vi "Sequencer Main.vi"() -> ()   [LabVIEW 2018] (continued)
                                n2343 = To Lower Case(string=w4629) -> (all lower case string=w4628:string)
                              }
                              n2344 = Multiply(x=w4617, y=-0.2) -> (x*y=w4620:dbl)
                              n2345 = Bundle("Lower Limit"=w4617, "Upper Limit"=w4618, "Numeric Value"=w4625) -> (w4626:T36)  [unwired: 1 in]
                              n2346 = Multiply(x=w4618, y=0.2) -> (x*y=w4622:dbl)
                              n2347 = Add(x=w4620, y=w4617) -> (x+y=w4619:dbl)
                              n2348 = Add(x=w4622, y=w4618) -> (x+y=w4621:dbl)
                              n2349 = property on="Limits" class="Slide (strict)"("Value"=w4626) -> ()  [unwired: 2 in, 2 out]
                              n2350 = property on="Limits" class="Slide (strict)"("Scale.Maximum"=w4621, "Scale.Minimum"=w4619) -> ()  [unwired: 2 in, 2 out]
                              n2351 = Index Array(array=w4615, index #1=0 ("index"), index #2=1 ("index"), index #3=2 ("index"), index #4=3 ("index"), index #5=4 ("index")) -> (element #1=w4614:string, element #2=w4608:string, element #3=w4607:string, element #4=w4606:string, element #5=w4605:string)
                            }
                            frame #1 {
                              n2352 = Not Equal?(x=w4648, y=4) -> (x != y?=w4640:bool)
                              n2353 = case shown="\"on\"" w4653 {
                                tunnel: w4652 -> [_ w4673]
                                tunnel: w4651 -> [_ w4672]
                                tunnel: w4650 -> [_ w4671]
                                tunnel: w4649 -> [_ w4670]
                                tunnel: [10000.0 w4661] -> w4642
                                tunnel: [w4655 w4660] -> w4646
                                tunnel: [w4654 w4659] -> w4645
                                tunnel: [w4654 w4658] -> w4644
                                tunnel: w4640 -> [_ w4657]
                                frame "off", Default {
                                w4654 = 0
                                w4655 = i16 0 items=["Sine"=0, "Square"=1, "Triangle"=2, "Ramp Up"=3, "Ramp Down"=4, "DC"=8, "Arbitrary"=6] ("Wave Type")
                                }
                                frame "on" {
                                w4664 = 1000000
                                n2354 = case shown="True" w4657 {
                                frame False {
                                }
                                frame True {
                                n2355 = One Button Dialog(message="PICo Scoê parameters\nErr!") -> ()  [unwired: 1 in, 1 out]
                                }
                                }
                                n2356 = Scan From String(input string=w4672) -> (output 1=w4667:dbl)  [unwired: 4 in, 3 out]
                                n2357 = Scan From String(input string=w4671) -> (output 1=w4666:dbl)  [unwired: 4 in, 3 out]
                                n2358 = Scan From String(input string=w4670) -> (output 1=w4665:dbl)  [unwired: 4 in, 3 out]
                                n2359 = Multiply(x=w4666, y=w4664) -> (x*y=w4663:dbl)
                                n2360 = Multiply(x=w4665, y=w4664) -> (x*y=w4662:dbl)
                                n2361 = To Long Integer(number=w4663) -> (32bit integer=w4659:i32)
                                n2362 = To Long Integer(number=w4662) -> (32bit integer=w4658:i32)
                                n2363 = case shown="\"triangle\"" w4673 {
                                tunnel: [w4677 w4678 w4679 w4680] -> w4660
                                frame "sine", Default {
                                w4677 = i16 0 items=["Sine"=0, "Square"=1, "Triangle"=2, "Ramp Up"=3, "Ramp Down"=4, "DC"=8, "Arbitrary"=6] ("Wave Type")
                                }
                                frame "square" {
                                w4678 = i16 1 items=["Sine"=0, "Square"=1, "Triangle"=2, "Ramp Up"=3, "Ramp Down"=4, "DC"=8, "Arbitrary"=6] ("Wave Type")
                                }
                                frame "triangle" {
                                w4679 = i16 2 items=["Sine"=0, "Square"=1, "Triangle"=2, "Ramp Up"=3, "Ramp Down"=4, "DC"=8, "Arbitrary"=6] ("Wave Type")
                                }
                                frame "dc" {
                                w4680 = i16 8 items=["Sine"=0, "Square"=1, "Triangle"=2, "Ramp Up"=3, "Ramp Down"=4, "DC"=8, "Arbitrary"=6] ("Wave Type")
                                }
                                }
                                n2364 = Greater Or Equal?(x=w4667, y=50000.0) -> (x >= y?=w4668:bool)
                                n2365 = case shown="True" w4668 {
                                tunnel: [w4675 50000.0] -> w4661
                                tunnel: w4667 -> [w4675 _]
                                frame False {
                                }
                                frame True {
                                }
                                }
                                }
                              }
                              n2366 = Bundle By Name(cluster=T29 {"Peak-to-Peak Voltage (microvolts)"=1000000, "Offset Voltage (microvolts)"=0, "Wave Type"=0, "Sweep Type"=0, "Shots"=0, "Sweeps"=0, "Trigger Type"=0, "Trigger Source"=0, "Ext. Threshold (ADC count)"=0, "White Noise"=FALSE} ("General AWG Settings"), "Wave Type"=w4646, "Peak-to-Peak Voltage (microvolts)"=w4645, "Offset Voltage (microvolts)"=w4644) -> (w4637:T29)
                              n2367 = global read "Global Variable.vi" "PicoScope Handle"() -> (w4638:u32)
                              n2368 = Bundle By Name(cluster=T30 {"Start Frequency"=1000.0, "Stop Frequency"=1000.0, "Increment"=0.0, "Dwell Time (seconds)"=0.0} ("Standard Waveform Settings"), "Start Frequency"=w4642, "Stop Frequency"=w4642) -> (w4639:T30)
                              n2369 = call "PicoScope3000aAWG.vi"("Standard Waveform Settings"=w4639, "General AWG Settings"=w4637, "Handle In"=w4638) -> ("error out"=w4636:errorcluster)  [unwired: 5 in, 3 out]
                              n2370 = call "PicoErrorHandler.vi"("error in"=w4636) -> ("error out"=w4635:errorcluster)
                              n2371 = call <userlib>:"Clear All Errors__ogtk.vi"("Error In"=w4635) -> ()  [unwired: 3 in, 1 out]
                            }
                          }
                          n2372 = Unbundle By Name(w4586) -> ("status"=w4584:bool)
                          n2373 = Not(x=w4584) -> (.not. x?=w4585:bool)
                          n2374 = case shown="True" w4585 {
                            tunnel: [enum16{"Idle", "PASS", "FALSE"}."FALSE" ("Step Test Result") enum16{"Idle", "PASS", "FALSE"}."PASS" ("Step Test Result")] -> w4592
                            frame False {
                            }
                            frame True {
                            }
                          }
                        }
                        frame 60 {
                          w4697 = "------------------------" ("string")
                          w4696 = "\r\n"
                          # "Step TEST Result"
                          # "Step Result Msg"
                          # "Str with \"false\" goto parameters"
                          # "Str \"false\" Preset"
                          # "Cmd Case"
                          # "Cmd Case"
                          n2375 = Unbundle By Name(w4710) -> ("Parameters"=w4692:string, "Step Description"=w4681:string, "Test Values.Numeric Value"=w4686:dbl, "Test Values.Upper Limit"=w4685:dbl, "Test Values.Lower Limit"=w4684:dbl)
                          n2376 = in-place {
                            in-place-border: w4692 -> [w4742]
                            in-place-border: [w4741] -> w4691
                            in-place-border: [w4740] -> w4689
                            # "STr \"fase\" exist"
                            n2377 = To Lower Case(string=w4742) -> (all lower case string=w4743:string)
                            n2378 = Match Pattern(string=w4743, regular expression="false") -> (after substring=w4745:string, offset past match=w4746:i32)  [unwired: 1 in, 2 out]
                            n2379 = Greater Or Equal To 0?(x=w4746) -> (x >= 0?=w4740:bool)
                            n2380 = case shown="True" w4740 {
                              tunnel: w4745 -> [_ w4749]
                              tunnel: [string[] [] w4748] -> w4741
                              frame False {
                                (unwired) ""
                              }
                              frame True {
                                n2381 = while {
                                shift-right: [w4753] -> _
                                shift-left: w4749 -> [w4754]
                                tunnel: [w4750] -> w4748 mode=indexing
                                stop <- w4752 stop-if-true
                                # "Get Array of Sub Parametrs"
                                n2382 = Match Pattern(string=w4754, regular expression=":") -> (before substring=w4750:string, after substring=w4753:string, offset past match=w4751:i32)  [unwired: 1 in, 1 out]
                                n2383 = Less Than 0?(x=w4751) -> (x < 0?=w4752:bool)
                                }
                              }
                            }
                          }
                          n2384 = while {
                            shift-right: [w4759] -> _
                            shift-left: w4692 -> [w4760]
                            tunnel: [w4756] -> w4694 mode=indexing
                            stop <- w4758 stop-if-true
                            # "Get Array of Parametrs"
                            n2385 = Match Pattern(string=w4760, regular expression=">") -> (before substring=w4756:string, after substring=w4759:string, offset past match=w4757:i32)  [unwired: 1 in, 1 out]
                            n2386 = Less Than 0?(x=w4757) -> (x < 0?=w4758:bool)
                          }
                          n2387 = Concatenate Strings(w4681, w4696, w4697, w4697, w4697, w4696) -> (w4698:string)
                          n2388 = property on="Tab Control Msg" class="TabCtl (strict)"("Value"=T21."Serial" ("Tab Control Msg")) -> (error out=w4708:errorcluster)  [unwired: 2 in, 1 out]
                          n2389 = property on="Serial CMD Mon" class="Str"("Value"=w4698) -> ()  [unwired: 2 in, 2 out]
                          n2390 = Index Array(array=w4694, index=0) -> (element=w4706:string)
                          n2391 = Index Array(array=w4694, index=1) -> (element=w4704:string)
                          n2392 = Index Array(array=w4694, index=2) -> (element=w4701:string)
                          n2393 = Index Array(array=w4694, index=3) -> (element=w4699:string)
                          n2394 = Index Array(array=w4694, index=4) -> (element=w4693:string)
                          n2395 = case shown="\"enable_ble\"" w4706 {
                            tunnel: w4708 -> [_ _ _ _ _ _ _ _ _ _ _ _ _ _ _ _ _ _ _ _]
                            tunnel: [enum16{"Idle", "PASS", "FALSE"}."FALSE" ("Step Test Result") w4770 w4814 w4842 w4885 w4935 w5079 w5119 w5165 w5343 w5414 w5573 w5623 w5672 w5708 w5745 w5782 w5814 w5846 w5878] -> w4707
                            tunnel: w4704 -> [_ w4768 _ _ _ w4947 w5083 w5117 _ w5341 w5440 _ _ w5673 _ w5746 _ _ w5844 _]
                            tunnel: w4701 -> [_ _ _ _ _ w4946 w5082 _ _ w5329 w5439 _ _ _ _ _ _ _ _ _]
                            tunnel: w4699 -> [_ _ _ _ _ w4945 w5081 _ _ _ _ _ _ _ _ _ _ _ _ _]
                            tunnel: w4693 -> [_ _ _ _ _ w4944 w5080 _ _ _ _ _ _ _ _ _ _ _ _ _]
                            tunnel: ["" w4767 w4811 w4840 w4876 w4934 w5078 w5115 w5163 w5328 w5434 "Set capmem '1' then '0' " w5622 w5671 _ _ w5780 w5812 _ _] -> w4683
                            tunnel: w4686 -> [_ _ _ _ _ _ _ _ _ _ _ _ _ _ _ _ _ _ _ _]
                            tunnel: w4685 -> [_ _ _ _ _ _ _ _ _ _ _ _ w5629 _ _ _ _ _ _ _]
                            tunnel: w4684 -> [_ _ _ _ _ _ _ _ _ _ _ _ w5628 _ _ _ _ _ _ _]
                            tunnel: ["" w4766 w4813 w4839 w4875 w4933 w5077 w5114 w5162 w5320 w5413 w5571 w5620 w5670 w5707 w5744 w5779 w5811 w5843 w5877] -> w4682
                            frame "False", Default {
                              n2396 = One Button Dialog(message="!Sequencer File Err") -> ()  [unwired: 1 in, 1 out]
                            }
                            frame "open" {
                              # "Param"
                              # "Cmd"
                              n2397 = flat-sequence {
                                tunnel: [w4782] -> w4772
                                tunnel: [w4781] -> w4771
                                tunnel: [w4780] -> w4769
                                tunnel: w4772 -> [w4788]
                                tunnel: w4771 -> [w4793]
                                tunnel: [w4794] -> w4770
                                tunnel: w4769 -> [w4791]
                                tunnel: w4768 -> [w4790]
                                tunnel: [w4792] -> w4767
                                tunnel: [w4791] -> w4766
                                frame #0 {
                                w4773 = u16 2 items=["None", "XON/XOFF", "RTS/CTS", "XON/XOFF & RTS/CTS", "DTR/DSR", "XON/XOFF & DTR/DSR"] ("flow control (0:none)")
                                n2398 = global read "Global Variable.vi" "COM Port FTDI RS232"() -> (w4779:refnum<visa-resource-name>)
                                n2399 = call "ADB-Serial_WrRd.vi"("flow control (0:none)"=w4773, "Tx Deay"=u16 5, "Timeout(Sec)"=2.0, "PassString"="Chuck(1)", "Command"="open", "ComPort"=w4779) -> ("error out"=w4781:errorcluster, "PASS"=w4782:bool, "received"=w4780:string)  [unwired: 3 in]
                                n2400 = invoke on="Serial CMD Mon" class="Str" method="Append String"("string"=w4780) -> ()  [unwired: 3 in, 4 out]
                                n2401 = Wait (ms)(milliseconds to wait=u32 500) -> ()  [unwired: 1 out]
                                }
                                frame #1 {
                                n2402 = String Length(string=w4790) -> (length=w4789:i32)
                                n2403 = Equal To 0?(x=w4789) -> (x = 0?=w4784:bool)
                                n2404 = Not(x=w4784) -> (.not. x?=w4783:bool)
                                n2405 = case shown="True" w4788 {
                                tunnel: w4791 -> [_ w4803]
                                tunnel: w4790 -> [_ w4807]
                                tunnel: [FALSE w4804] -> w4786
                                tunnel: ["!Firmware vertion not Right" ("line") w4802] -> w4792
                                frame False {
                                }
                                frame True {
                                n2406 = To Lower Case(string=w4807) -> (all lower case string=w4806:string)
                                n2407 = To Lower Case(string=w4803) -> (all lower case string=w4808:string)
                                n2408 = Match Pattern(string=w4808, regular expression=w4806) -> (match substring=w4800:string, offset past match=w4805:i32)  [unwired: 1 in, 2 out]
                                n2409 = Greater Than 0?(x=w4805) -> (x > 0?=w4804:bool)
                                n2410 = Concatenate Strings("version: ", w4800) -> (w4802:string)
                                }
                                }
                                n2411 = And(x=w4788, y=w4784) -> (x .and. y?=w4785:bool)
                                n2412 = global read "Global Variable.vi" "Array Errors"() -> (w4797:errorcluster[])
                                n2413 = Replace Array Subset(array=w4797, new element=w4793, index=3) -> (w4796:errorcluster[])
                                n2414 = global write "Global Variable.vi" "Array Errors"(w4796) -> ()
                                n2415 = Select(t=w4786, s=w4783, f=w4785) -> (s? t:f=w4787:bool)
                                n2416 = case shown="True" w4787 {
                                tunnel: [enum16{"Idle", "PASS", "FALSE"}."FALSE" ("Step Test Result") enum16{"Idle", "PASS", "FALSE"}."PASS" ("Step Test Result")] -> w4794
                                frame False {
                                # "Step TEST Result"
                                }
                                frame True {
                                # "Step TEST Result"
                                }
                                }
                                }
                              }
                            }
                            frame "passwd" {
                              n2417 = flat-sequence {
                                tunnel: [w4826] -> w4816
                                tunnel: [w4825] -> w4815
                                tunnel: [w4824] -> w4812
                                tunnel: w4816 -> [w4829]
                                tunnel: w4815 -> [w4830]
                                tunnel: [w4831] -> w4814
                                tunnel: [w4828] -> w4813
                                tunnel: w4812 -> [w4828]
                                tunnel: [w4827] -> w4811
                                frame #0 {
                                w4817 = u16 2 items=["None", "XON/XOFF", "RTS/CTS", "XON/XOFF & RTS/CTS", "DTR/DSR", "XON/XOFF & DTR/DSR"] ("flow control (0:none)")
                                n2418 = global read "Global Variable.vi" "COM Port FTDI RS232"() -> (w4823:refnum<visa-resource-name>)
                                n2419 = call "ADB-Serial_WrRd.vi"("flow control (0:none)"=w4817, "Tx Deay"=u16 5, "Timeout(Sec)"=2.0, "PassString"="Chuck(3)", "Command"="passwd admin", "ComPort"=w4823) -> ("error out"=w4825:errorcluster, "PASS"=w4826:bool, "received"=w4824:string)  [unwired: 3 in]
                                n2420 = invoke on="Serial CMD Mon" class="Str" method="Append String"("string"=w4824) -> ()  [unwired: 3 in, 4 out]
                                n2421 = Wait (ms)(milliseconds to wait=u32 250) -> ()  [unwired: 1 out]
                                }
                                frame #1 {
                                n2422 = global read "Global Variable.vi" "Array Errors"() -> (w4834:errorcluster[])
                                n2423 = case shown="False" w4829 {
                                tunnel: [enum16{"Idle", "PASS", "FALSE"}."FALSE" ("Step Test Result") enum16{"Idle", "PASS", "FALSE"}."PASS" ("Step Test Result")] -> w4831
                                tunnel: ["Err" "Admin"] -> w4827
                                frame False {
                                # "Step TEST Result"
                                }
                                frame True {
                                # "Step TEST Result"
                                }
                                }
                                n2424 = Replace Array Subset(array=w4834, new element=w4830, index=3) -> (w4833:errorcluster[])
                                n2425 = global write "Global Variable.vi" "Array Errors"(w4833) -> ()
                                }
                              }
                            }
                            frame "getpid" {
                              # "Param"
                              # "Cmd"
                              n2426 = flat-sequence {
                                tunnel: [w4854] -> w4844
                                tunnel: [w4853] -> w4843
                                tunnel: [w4852] -> w4841
                                tunnel: [w4852] -> _
                                tunnel: [w4852] -> w4839
                                tunnel: w4844 -> [w4858]
                                tunnel: w4843 -> [w4861]
                                tunnel: [w4862] -> w4842
                                tunnel: [w4855] -> w4840
                                tunnel: w4841 -> [w4859]
                                frame #0 {
                                w4845 = u16 2 items=["None", "XON/XOFF", "RTS/CTS", "XON/XOFF & RTS/CTS", "DTR/DSR", "XON/XOFF & DTR/DSR"] ("flow control (0:none)")
                                n2427 = global read "Global Variable.vi" "COM Port FTDI RS232"() -> (w4851:refnum<visa-resource-name>)
                                n2428 = global read "Global Variable.vi" "Wr PID"() -> (w4848:string)
                                n2429 = call "ADB-Serial_WrRd.vi"("flow control (0:none)"=w4845, "Tx Deay"=u16 5, "Timeout(Sec)"=2.0, "PassString"=w4848, "Command"="getPID", "ComPort"=w4851) -> ("error out"=w4853:errorcluster, "PASS"=w4854:bool, "received"=w4852:string)  [unwired: 3 in]
                                n2430 = invoke on="Serial CMD Mon" class="Str" method="Append String"("string"=w4852) -> ()  [unwired: 3 in, 4 out]
                                n2431 = Wait (ms)(milliseconds to wait=u32 250) -> ()  [unwired: 1 out]
                                }
                                frame #1 {
                                n2432 = in-place {
                                in-place-border: w4861 -> [w4869]
                                in-place-border: [w4869] -> w4860
                                in-place-border: [w4870] -> w4856
                                in-place-border: w4859 -> [w4867]
                                n2433 = Match Pattern(string=w4867, regular expression="PID:" ("search string/char (-)")) -> (after substring=w4866:string)  [unwired: 1 in, 3 out]
                                n2434 = String Subset(string=w4866, offset (0)=1, length (rest)=13 ("length (rest)")) -> (substring=w4870:string)
                                n2435 = global write "Global Variable.vi" "Rd PID"(w4870) -> ()
                                }
                                n2436 = global read "Global Variable.vi" "Array Errors"() -> (w4865:errorcluster[])
                                n2437 = case shown="False" w4858 {
                                tunnel: [enum16{"Idle", "PASS", "FALSE"}."FALSE" ("Step Test Result") enum16{"Idle", "PASS", "FALSE"}."PASS" ("Step Test Result")] -> w4862
                                frame False {
                                # "Step TEST Result"
                                }
                                frame True {
                                # "Step TEST Result"
                                }
                                }
                                n2438 = Replace Array Subset(array=w4865, new element=w4860, index=3) -> (w4864:errorcluster[])
                                n2439 = global write "Global Variable.vi" "Array Errors"(w4864) -> ()
                                n2440 = Concatenate Strings("Read PID: " ("string"), w4856) -> (w4855:string)
                                }
                              }
                            }
                            frame "setpid" {
                              n2441 = flat-sequence {
                                tunnel: [w4888] -> w4879
                                tunnel: [w4930] -> w4881
                                tunnel: [w4929] -> w4880
                                tunnel: w4879 -> [w4924]
                                tunnel: [w4926] -> w4877
                                tunnel: [w4925] -> w4875
                                frame #0 {
                                w4899 = 5
                                # "Replace Space to 0"
                                # "YY: Year 00-99\nWW: Week 01-53\nSS: Supplier ID (SVI: 04)\nxx: Spare\nNNNNN: Ser Number"
                                # "default"
                                n2442 = local read "Barcode"() -> (w4887:string)
                                n2443 = global write "Global Variable.vi" "Wr PID"("") -> ()
                                n2444 = String Length(string=w4887) -> (length=w4898:i32)
                                n2445 = Greater?(x=w4898, y=w4899) -> (0:w4900:bool)
                                n2446 = case shown="True" w4900 {
                                tunnel: w4887 -> [_ w4923]
                                tunnel: w4899 -> [_ w4921]
                                tunnel: w4898 -> [_ w4922]
                                tunnel: "1111040011111" ("ADB_PID") -> [w4903 w4919]
                                tunnel: [w4903 w4909] -> w4893
                                frame False {
                                }
                                frame True {
                                w4905 = "%2d" ("format string")
                                n2447 = Subtract(x=w4922, y=w4921) -> (x-y=w4920:i32)
                                n2448 = call "Calc_ISO_WeekNumber.vi"() -> ("ISO week number"=w4904:i32, "SBZ year 2 digits"=w4908:i32)  [unwired: 5 in, 5 out]
                                n2449 = String Subset(string=w4923, offset (0)=w4920, length (rest)=w4921) -> (substring=w4918:string)
                                n2450 = Format Into String(format string=w4905, w4908) -> (resulting string=w4907:string)  [unwired: 2 in, 1 out]
                                n2451 = Replace Substring(2:5 ("length (len. of substring)"), 3:8 ("offset (0)"), 4:w4918, 5:w4919) -> (1:w4915:string)  [unwired: 1 out]
                                n2452 = Format Into String(format string=w4905, w4904) -> (resulting string=w4906:string)  [unwired: 2 in, 1 out]
                                n2453 = Replace Substring(2:2 ("offset (0)"), 3:0 ("offset (0)"), 4:w4907, 5:w4915) -> (1:w4910:string)  [unwired: 1 out]
                                n2454 = Replace Substring(2:2 ("offset (0)"), 3:2 ("offset (0)"), 4:w4906, 5:w4910) -> (1:w4909:string)  [unwired: 1 out]
                                }
                                }
                                n2455 = local read "Barcode\nDefault"() -> (w4886:bool)
                                n2456 = call <vilib>:"Space Constant.vi"() -> ("String"=w4891:string)
                                n2457 = call <vilib>:"Search and Replace Pattern.vi"("string"=w4893, "regular expression (\"\")"=w4891, "replace string (\"\")"="0" ("replace string (\"\")")) -> ("result string"=w4889:string)  [unwired: 2 in, 1 out]
                                n2458 = case shown="False" w4886 {
                                tunnel: w4889 -> [_ w4902]
                                tunnel: [w4901 w4902] -> w4888
                                tunnel: w4887 -> [w4901 _]
                                frame False {
                                }
                                frame True {
                                }
                                }
                                n2459 = Concatenate Strings("Calculated PID: ", w4888, "\r\n") -> (w4890:string)
                                n2460 = invoke on="Serial CMD Mon" class="Str" method="Append String"("string"=w4890) -> ()  [unwired: 3 in, 4 out]
                                }
                                frame #1 {
                                n2461 = global read "Global Variable.vi" "COM Port FTDI RS232"() -> (w4928:refnum<visa-resource-name>)
                                n2462 = call "ADB-SetPID.vi"("ADB_PID"=w4924, "ComPort"=w4928) -> ("error out"=w4929:errorcluster, "Wr PID"=w4926:string, "PASS"=w4930:bool, "received"=w4925:string)  [unwired: 6 in]
                                n2463 = invoke on="Serial CMD Mon" class="Str" method="Append String"("string"=w4925) -> ()  [unwired: 3 in, 4 out]
                                n2464 = global write "Global Variable.vi" "Wr PID"(w4926) -> ()
                                n2465 = Wait (ms)(milliseconds to wait=u32 5000) -> ()  [unwired: 1 out]
                                }
                              }
                              n2466 = global read "Global Variable.vi" "Array Errors"() -> (w4884:errorcluster[])
                              n2467 = case shown="False" w4881 {
                                tunnel: [enum16{"Idle", "PASS", "FALSE"}."FALSE" ("Step Test Result") enum16{"Idle", "PASS", "FALSE"}."PASS" ("Step Test Result")] -> w4885
                                frame False {
                                # "Step TEST Result"
                                }
                                frame True {
                                # "Step TEST Result"
                                }
                              }
                              n2468 = Replace Array Subset(array=w4884, new element=w4880, index=5) -> (w4883:errorcluster[])
                              n2469 = Concatenate Strings("Write PID: " ("string"), w4877) -> (w4876:string)
                              n2470 = global write "Global Variable.vi" "Array Errors"(w4883) -> ()
                            }
                            frame "recvtest" {
                              # "Param 1-4"
                              # "Cmd"
                              n2471 = flat-sequence {
                                tunnel: [w4966] -> w4950
                                tunnel: [w4965] -> w4949
                                tunnel: [w4964] -> w4948
                                tunnel: w4947 -> [w4963]
                                tunnel: w4946 -> [w4962]
                                tunnel: w4945 -> [w4961]
                                tunnel: w4944 -> [w4960]
                                tunnel: [w4959] -> w4943
                                tunnel: [w4958] -> w4942
                                tunnel: [w4957] -> w4941
                                tunnel: [w4956] -> w4940
                                tunnel: [w4955] -> w4939
                                tunnel: [w4954] -> w4938
                                tunnel: [w4953] -> w4937
                                tunnel: [w4952] -> w4936
                                tunnel: w4950 -> [w5005]
                                tunnel: w4949 -> [w5024]
                                tunnel: [w5025] -> w4935
                                tunnel: w4948 -> [w5003]
                                tunnel: w4943 -> [w5015]
                                tunnel: w4942 -> [w5014]
                                tunnel: w4941 -> [w5013]
                                tunnel: w4940 -> [w5012]
                                tunnel: w4939 -> [w5011]
                                tunnel: w4938 -> [w5010]
                                tunnel: w4937 -> [w5009]
                                tunnel: w4936 -> [w5008]
                                tunnel: [w5004] -> w4934
                                tunnel: [w5003] -> w4933
                                frame #0 {
                                w4951 = "%f" ("format string")
                                n2472 = for {
                                N: 1 -> [_]
                                tunnel: [w4999] -> w4966
                                tunnel: [w4998] -> w4965
                                tunnel: [w4997] -> w4964
                                stop <- w4999 stop-if-true
                                n2473 = global read "Global Variable.vi" "COM Port FTDI RS232"() -> (w5002:refnum<visa-resource-name>)
                                n2474 = call "ADB-Serial_WrRd.vi"("Timeout(Sec)"=5.0, "PassString"="Chuck(3):", "Command"="recvtest", "ComPort"=w5002) -> ("error out"=w4998:errorcluster, "PASS"=w4999:bool, "received"=w4997:string)  [unwired: 5 in]
                                n2475 = invoke on="Serial CMD Mon" class="Str" method="Append String"("string"=w4997) -> ()  [unwired: 3 in, 4 out]
                                }
                                n2476 = in-place {
                                in-place-border: w4963 -> [w4995]
                                in-place-border: [w4991] -> w4959
                                in-place-border: [w4990] -> w4958
                                in-place-border: w4951 -> [w4989]
                                # "max"
                                # "min"
                                # "LMS RX -> k_est"
                                n2477 = Match Pattern(string=w4995, regular expression=":") -> (before substring=w4993:string, after substring=w4992:string)  [unwired: 1 in, 2 out]
                                n2478 = Scan From String(format string=w4989, input string=w4993) -> (output 1=w4991:dbl)  [unwired: 3 in, 3 out]
                                n2479 = Scan From String(format string=w4989, input string=w4992) -> (output 1=w4990:dbl)  [unwired: 3 in, 3 out]
                                }
                                n2480 = in-place {
                                in-place-border: w4962 -> [w4988]
                                in-place-border: [w4984] -> w4957
                                in-place-border: [w4983] -> w4956
                                in-place-border: w4951 -> [w4982]
                                # "max"
                                # "min"
                                # "LMS RX -> I_est"
                                n2481 = Match Pattern(string=w4988, regular expression=":") -> (before substring=w4986:string, after substring=w4985:string)  [unwired: 1 in, 2 out]
                                n2482 = Scan From String(format string=w4982, input string=w4986) -> (output 1=w4984:dbl)  [unwired: 3 in, 3 out]
                                n2483 = Scan From String(format string=w4982, input string=w4985) -> (output 1=w4983:dbl)  [unwired: 3 in, 3 out]
                                }
                                n2484 = in-place {
                                in-place-border: w4961 -> [w4981]
                                in-place-border: [w4977] -> w4955
                                in-place-border: [w4976] -> w4954
                                in-place-border: w4951 -> [w4975]
                                # "max"
                                # "min"
                                # "CURRENT -> k_est"
                                n2485 = Match Pattern(string=w4981, regular expression=":") -> (before substring=w4979:string, after substring=w4978:string)  [unwired: 1 in, 2 out]
                                n2486 = Scan From String(format string=w4975, input string=w4979) -> (output 1=w4977:dbl)  [unwired: 3 in, 3 out]
                                n2487 = Scan From String(format string=w4975, input string=w4978) -> (output 1=w4976:dbl)  [unwired: 3 in, 3 out]
                                }
                                n2488 = in-place {
                                in-place-border: w4960 -> [w4974]
                                in-place-border: [w4971] -> w4953
                                in-place-border: [w4970] -> w4952
                                in-place-border: w4951 -> [w4969]
                                # "max"
                                # "min"
                                # "CURRENT -> I_est"
                                n2489 = Match Pattern(string=w4974, regular expression=":") -> (before substring=w4973:string, after substring=w4972:string)  [unwired: 1 in, 2 out]
                                n2490 = Scan From String(format string=w4969, input string=w4973) -> (output 1=w4971:dbl)  [unwired: 3 in, 3 out]
                                n2491 = Scan From String(format string=w4969, input string=w4972) -> (output 1=w4970:dbl)  [unwired: 3 in, 3 out]
                                }
                                }
                                frame #1 {
                                n2492 = Match Pattern(string=w5003, regular expression="CURRENT:") -> (after substring=w5006:string, offset past match=w5020:i32)  [unwired: 1 in, 2 out]
                                n2493 = Match Pattern(string=w5003, regular expression="LMS_RX:") -> (after substring=w5007:string, offset past match=w5021:i32)  [unwired: 1 in, 2 out]
                                n2494 = Greater Than 0?(x=w5021) -> (x > 0?=w5018:bool)
                                n2495 = Greater Than 0?(x=w5020) -> (x > 0?=w5019:bool)
                                n2496 = Compound Arithmetic op=AND(w5018, w5019, w5005) -> (w5017:bool)
                                n2497 = case shown="True" w5017 {
                                tunnel: [FALSE w5060] -> w5016
                                tunnel: w5015 -> [_ w5070]
                                tunnel: w5014 -> [_ w5069]
                                tunnel: w5013 -> [_ w5067]
                                tunnel: w5012 -> [_ w5068]
                                tunnel: w5011 -> [_ w5065]
                                tunnel: w5010 -> [_ w5064]
                                tunnel: w5009 -> [_ w5063]
                                tunnel: w5008 -> [_ w5062]
                                tunnel: w5006 -> [_ w5055]
                                tunnel: w5007 -> [_ w5054]
                                tunnel: ["" w5048] -> w5004
                                frame False {
                                }
                                frame True {
                                w5032 = ":" ("string")
                                n2498 = Match Pattern(string=w5054, regular expression="k_est") -> (after substring=w5053:string)  [unwired: 1 in, 3 out]
                                n2499 = Match Pattern(string=w5054, regular expression="l_est") -> (after substring=w5066:string)  [unwired: 1 in, 3 out]
                                n2500 = Match Pattern(string=w5055, regular expression="k_est") -> (after substring=w5041:string)  [unwired: 1 in, 3 out]
                                n2501 = Match Pattern(string=w5055, regular expression="l_est") -> (after substring=w5061:string)  [unwired: 1 in, 3 out]
                                n2502 = call <userlib>:"Multi-line String to Array__ogtk.vi"("string"=w5053) -> ("lines"=w5052:string[])
                                n2503 = call "Loop Test.vi"("Min"=w5070, "Max"=w5069, "Data Str"=w5053) -> ("Result"=w5059:bool)  [unwired: 8 in]
                                n2504 = call "Loop Test.vi"("Min"=w5067, "Max"=w5068, "Data Str"=w5066) -> ("Result"=w5058:bool)  [unwired: 8 in]
                                n2505 = call "Loop Test.vi"("Min"=w5065, "Max"=w5064, "Data Str"=w5041) -> ("Result"=w5057:bool)  [unwired: 8 in]
                                n2506 = call "Loop Test.vi"("Min"=w5063, "Max"=w5062, "Data Str"=w5061) -> ("Result"=w5056:bool)  [unwired: 8 in]
                                n2507 = call <userlib>:"Multi-line String to Array__ogtk.vi"("string"=w5041) -> ("lines"=w5038:string[])
                                n2508 = Index Array(array=w5052, index #1=0, index #2=1) -> (element #1=w5046:string, element #2=w5043:string)
                                n2509 = Index Array(array=w5038, index #1=0, index #2=1) -> (element #1=w5037:string, element #2=w5036:string)
                                n2510 = Compound Arithmetic op=AND(w5059, w5058, w5057, w5056) -> (w5060:bool)
                                n2511 = String Subset(string=w5046, offset (0)=2) -> (substring=w5047:string)  [unwired: 1 in]
                                n2512 = String Subset(string=w5043, offset (0)=7) -> (substring=w5044:string)  [unwired: 1 in]
                                n2513 = String Subset(string=w5037, offset (0)=2) -> (substring=w5033:string)  [unwired: 1 in]
                                n2514 = String Subset(string=w5036, offset (0)=7) -> (substring=w5031:string)  [unwired: 1 in]
                                n2515 = Concatenate Strings(w5047, w5032, w5044, "\r\n", w5033, w5032, w5031) -> (w5048:string)
                                }
                                }
                                n2516 = global read "Global Variable.vi" "Array Errors"() -> (w5028:errorcluster[])
                                n2517 = Replace Array Subset(array=w5028, new element=w5024, index=3) -> (w5027:errorcluster[])
                                n2518 = case shown="False" w5016 {
                                tunnel: [enum16{"Idle", "PASS", "FALSE"}."FALSE" ("Step Test Result") enum16{"Idle", "PASS", "FALSE"}."PASS" ("Step Test Result")] -> w5025
                                frame False {
                                # "Step TEST Result"
                                }
                                frame True {
                                # "Step TEST Result"
                                }
                                }
                                n2519 = global write "Global Variable.vi" "Array Errors"(w5027) -> ()
                                }
                              }
                            }
                            frame "recvtest_2" {
                              # "Param 1-4"
                              # "Cmd"
                              n2520 = flat-sequence {
                                tunnel: [w5095] -> w5086
                                tunnel: [w5094] -> w5085
                                tunnel: [w5093] -> w5084
                                tunnel: w5083 -> [_]
                                tunnel: w5082 -> [_]
                                tunnel: w5081 -> [_]
                                tunnel: w5080 -> [_]
                                tunnel: w5086 -> [w5099]
                                tunnel: w5085 -> [w5100]
                                tunnel: [w5101] -> w5079
                                tunnel: w5084 -> [w5096]
                                tunnel: [w5097] -> w5078
                                tunnel: [w5096] -> w5077
                                frame #0 {
                                w5087 = u16 2 items=["None", "XON/XOFF", "RTS/CTS", "XON/XOFF & RTS/CTS", "DTR/DSR", "XON/XOFF & DTR/DSR"] ("flow control (0:none)")
                                n2521 = global read "Global Variable.vi" "COM Port FTDI RS232"() -> (w5092:refnum<visa-resource-name>)
                                n2522 = call "ADB-Serial_WrRd.vi"("flow control (0:none)"=w5087, "Tx Deay"=u16 5, "Timeout(Sec)"=5.0, "PassString"="Chuck(3):", "Command"="recvtest", "ComPort"=w5092) -> ("error out"=w5094:errorcluster, "PASS"=w5095:bool, "received"=w5093:string)  [unwired: 3 in]
                                n2523 = invoke on="Serial CMD Mon" class="Str" method="Append String"("string"=w5093) -> ()  [unwired: 3 in, 4 out]
                                }
                                frame #1 {
                                n2524 = case shown="True" w5099 {
                                tunnel: w5096 -> [_ w5111]
                                tunnel: [FALSE w5110] -> w5098
                                tunnel: ["Err" ("received") w5109] -> w5097
                                frame False {
                                }
                                frame True {
                                n2525 = Match Pattern(string=w5111, regular expression="TEST SUCCEED") -> (match substring=w5109:string, offset past match=w5108:i32)  [unwired: 1 in, 2 out]
                                n2526 = Greater Than 0?(x=w5108) -> (x > 0?=w5110:bool)
                                }
                                }
                                n2527 = global read "Global Variable.vi" "Array Errors"() -> (w5104:errorcluster[])
                                n2528 = case shown="True" w5098 {
                                tunnel: [enum16{"Idle", "PASS", "FALSE"}."FALSE" ("Step Test Result") enum16{"Idle", "PASS", "FALSE"}."PASS" ("Step Test Result")] -> w5101
                                frame False {
                                # "Step TEST Result"
                                }
                                frame True {
                                # "Step TEST Result"
                                }
                                }
                                n2529 = Replace Array Subset(array=w5104, new element=w5100, index=3) -> (w5103:errorcluster[])
                                n2530 = global write "Global Variable.vi" "Array Errors"(w5103) -> ()
                                }
                              }
                            }
                            frame "readcputemp" {
                              # "Param"
                              # "Cmd"
                              n2531 = flat-sequence {
                                tunnel: [w5130] -> w5120
                                tunnel: [w5128] -> w5118
                                tunnel: [w5129] -> w5116
                                tunnel: [w5128] -> w5114
                                tunnel: w5120 -> [w5140]
                                tunnel: [w5142] -> w5119
                                tunnel: w5118 -> [w5139]
                                tunnel: w5117 -> [w5138]
                                tunnel: w5116 -> [w5137]
                                tunnel: [w5132] -> w5115
                                frame #0 {
                                w5121 = u16 0 items=["None", "XON/XOFF", "RTS/CTS", "XON/XOFF & RTS/CTS", "DTR/DSR", "XON/XOFF & DTR/DSR"] ("flow control (0:none)")
                                n2532 = global read "Global Variable.vi" "COM Port FTDI RS232"() -> (w5127:refnum<visa-resource-name>)
                                n2533 = call "ADB-Serial_WrRd.vi"("flow control (0:none)"=w5121, "Tx Deay"=u16 5, "Timeout(Sec)"=2.0, "PassString"="Chuck(3)", "Command"="readcputemp", "ComPort"=w5127) -> ("error out"=w5129:errorcluster, "PASS"=w5130:bool, "received"=w5128:string)  [unwired: 3 in]
                                n2534 = invoke on="Serial CMD Mon" class="Str" method="Append String"("string"=w5128) -> ()  [unwired: 3 in, 4 out]
                                n2535 = Wait (ms)(milliseconds to wait=u32 300) -> ()  [unwired: 1 out]
                                }
                                frame #1 {
                                n2536 = case shown="True" w5140 {
                                tunnel: [FALSE w5157] -> w5141
                                tunnel: w5139 -> [_ w5154]
                                tunnel: w5138 -> [_ w5153]
                                tunnel: w5137 -> [w5147 w5151]
                                tunnel: [w5147 w5152] -> w5134
                                tunnel: [0.0 w5149] -> w5136
                                frame False {
                                }
                                frame True {
                                n2537 = Match Pattern(string=w5154, regular expression=w5153) -> (after substring=w5150:string)  [unwired: 1 in, 3 out]
                                n2538 = Scan From String(format string="%.; %.3f", input string=w5150, error in=w5151) -> (error out=w5152:errorcluster, output 1=w5149:dbl)  [unwired: 2 in, 2 out]
                                n2539 = Greater Than 0?(x=w5149) -> (x > 0?=w5155:bool)
                                n2540 = case shown="True" w5155 {
                                tunnel: [FALSE TRUE] -> w5157
                                frame False {
                                }
                                frame True {
                                }
                                }
                                }
                                }
                                n2541 = global read "Global Variable.vi" "Array Errors"() -> (w5145:errorcluster[])
                                n2542 = case shown="False" w5141 {
                                tunnel: [enum16{"Idle", "PASS", "FALSE"}."FALSE" ("Step Test Result") enum16{"Idle", "PASS", "FALSE"}."PASS" ("Step Test Result")] -> w5142
                                frame False {
                                # "Step TEST Result"
                                }
                                frame True {
                                # "Step TEST Result"
                                }
                                }
                                n2543 = Format Into String(format string="%.1f C°", initial string="CPU Temp: ", error in=w5134, w5136) -> (resulting string=w5132:string, error out=w5133:errorcluster)
                                n2544 = Replace Array Subset(array=w5145, new element=w5133, index=3) -> (w5144:errorcluster[])
                                n2545 = global write "Global Variable.vi" "Array Errors"(w5144) -> ()
                                }
                              }
                            }
                            frame "up" {
                              # "Param"
                              # "Cmd"
                              n2546 = flat-sequence {
                                tunnel: [w5176] -> w5167
                                tunnel: [w5175] -> w5166
                                tunnel: [w5174] -> w5164
                                tunnel: w5167 -> [w5179]
                                tunnel: w5166 -> [w5181]
                                tunnel: [w5182] -> w5165
                                tunnel: w5164 -> [w5177]
                                tunnel: [w5178] -> w5163
                                tunnel: [w5177] -> w5162
                                frame #0 {
                                w5168 = u16 2 items=["None", "XON/XOFF", "RTS/CTS", "XON/XOFF & RTS/CTS", "DTR/DSR", "XON/XOFF & DTR/DSR"] ("flow control (0:none)")
                                n2547 = global read "Global Variable.vi" "COM Port FTDI RS232"() -> (w5173:refnum<visa-resource-name>)
                                n2548 = call "ADB-Serial_WrRd.vi"("flow control (0:none)"=w5168, "Tx Deay"=u16 5, "Timeout(Sec)"=2.0, "PassString"="Totally", "Command"="up", "ComPort"=w5173) -> ("error out"=w5175:errorcluster, "PASS"=w5176:bool, "received"=w5174:string)  [unwired: 3 in]
                                n2549 = invoke on="Serial CMD Mon" class="Str" method="Append String"("string"=w5174) -> ()  [unwired: 3 in, 4 out]
                                }
                                frame #1 {
                                n2550 = case shown="True" w5179 {
                                tunnel: [FALSE w5195] -> w5180
                                tunnel: w5177 -> [_ w5189]
                                tunnel: ["" w5188] -> w5178
                                frame False {
                                }
                                frame True {
                                n2551 = Match Pattern(string=w5189, regular expression="Totally") -> (after substring=w5192:string)  [unwired: 1 in, 3 out]
                                n2552 = Scan From String(format string="%d", input string=w5192) -> (output 1=w5190:i32)  [unwired: 3 in, 3 out]
                                n2553 = Not Equal To 0?(x=w5190) -> (x != 0?=w5194:bool)
                                n2554 = case shown="True" w5194 {
                                tunnel: [FALSE TRUE] -> w5195
                                tunnel: w5189 -> [_ w5200]
                                tunnel: ["" w5198] -> w5188
                                frame False {
                                }
                                frame True {
                                n2555 = xnode "Match Regular Expression"("input string"=w5200, "regular expression"="\\((.*)\\)") -> ("submatch 1"=w5198:string)  [unwired: 4 in, 5 out]
                                }
                                }
                                }
                                }
                                n2556 = global read "Global Variable.vi" "Array Errors"() -> (w5185:errorcluster[])
                                n2557 = case shown="True" w5180 {
                                tunnel: [enum16{"Idle", "PASS", "FALSE"}."FALSE" ("Step Test Result") enum16{"Idle", "PASS", "FALSE"}."PASS" ("Step Test Result")] -> w5182
                                frame False {
                                # "Step TEST Result"
                                }
                                frame True {
                                # "Step TEST Result"
                                }
                                }
                                n2558 = Replace Array Subset(array=w5185, new element=w5181, index=3) -> (w5184:errorcluster[])
                                n2559 = global write "Global Variable.vi" "Array Errors"(w5184) -> ()
                                }
                              }
                            }
                            frame "readvolt" {
                              # "Param"
                              # "Cmd"
                              n2560 = flat-sequence {
                                tunnel: [w5369] -> w5345
                                tunnel: [w5368] -> w5344
                                tunnel: [w5367] -> w5342
                                tunnel: [w5367] -> w5320
                                tunnel: w5345 -> [w5387]
                                tunnel: w5344 -> [w5388]
                                tunnel: w5342 -> [w5370]
                                tunnel: w5341 -> [w5378]
                                tunnel: w5334 -> [w5386]
                                tunnel: w5335 -> [w5385]
                                tunnel: w5324 -> [w5372]
                                tunnel: w5323 -> [w5375]
                                tunnel: [w5371] -> w5327
                                tunnel: [w5389] -> w5322
                                tunnel: [w5371] -> w5321
                                tunnel: [w5411] -> w5328
                                tunnel: [w5412] -> w5343
                                tunnel: w5322 -> [w5412]
                                tunnel: w5321 -> [w5411]
                                frame #0 {
                                w5361 = u16 2 items=["None", "XON/XOFF", "RTS/CTS", "XON/XOFF & RTS/CTS", "DTR/DSR", "XON/XOFF & DTR/DSR"] ("flow control (0:none)")
                                n2561 = global read "Global Variable.vi" "COM Port FTDI RS232"() -> (w5366:refnum<visa-resource-name>)
                                n2562 = call "ADB-Serial_WrRd.vi"("flow control (0:none)"=w5361, "Tx Deay"=u16 5, "Timeout(Sec)"=2.0, "PassString"="Voltages", "Command"="readvolt", "ComPort"=w5366) -> ("error out"=w5368:errorcluster, "PASS"=w5369:bool, "received"=w5367:string)  [unwired: 3 in]
                                n2563 = invoke on="Serial CMD Mon" class="Str" method="Append String"("string"=w5367) -> ()  [unwired: 3 in, 4 out]
                                }
                                frame #1 {
                                w5380 = "\r\n"
                                w5373 = ">"
                                w5374 = "<"
                                w5382 = "\r\n"
                                w5381 = "******************************************" ("string")
                                n2564 = global read "Global Variable.vi" "Array Errors"() -> (w5392:errorcluster[])
                                n2565 = case shown="True" w5387 {
                                tunnel: w5370 -> [_ w5403]
                                tunnel: w5378 -> [_ w5399]
                                tunnel: w5386 -> [_ w5398]
                                tunnel: w5385 -> [_ w5397]
                                tunnel: [FALSE w5396] -> w5384
                                tunnel: [0 ("Numeric") w5395] -> w5383
                                frame False {
                                }
                                frame True {
                                n2566 = Match Pattern(string=w5403, regular expression=w5399) -> (after substring=w5401:string, offset past match=w5402:i32)  [unwired: 1 in, 2 out]
                                n2567 = Greater Than 0?(x=w5402) -> (x > 0?=w5400:bool)
                                n2568 = case shown="False" w5400 {
                                tunnel: w5401 -> [_ w5408]
                                tunnel: [-9999 ("Numeric") w5405] -> w5395
                                frame False {
                                }
